vi "Convert Params.vi"(11 "Experiment Parameter Values":T1(array[cluster])) -> (3 "Matlab Param Array":cluster{"Name":string, "Data":variant}[](array[cluster]))   [LabVIEW 2014, in "Matlab API.lvlib"]
uses:
  Matlab API.lvlib
  <vilib>/Utility/error.llb/DialogType.ctl
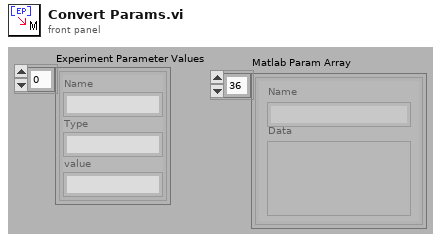
[diagram p1: front panel]
types:
  T1 = cluster{"Name":string, "Type":string, "value":string}[]
  T2 = typedef "DialogType.ctl" = u16
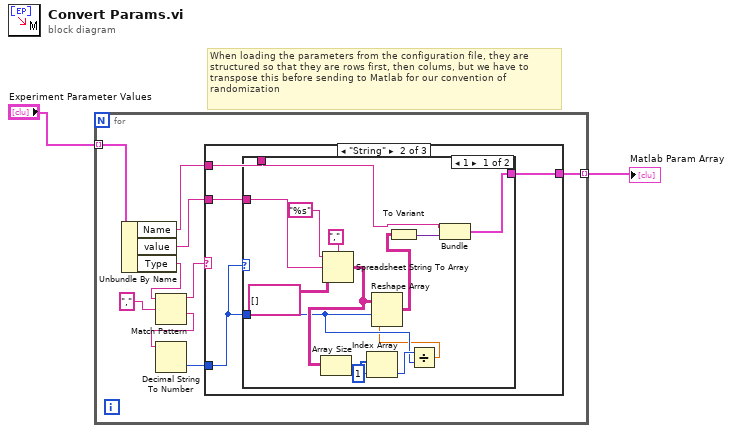
[diagram p0: block diagram]
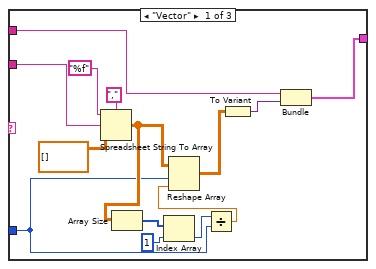
[diagram p2: hidden frame]
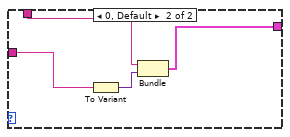
[diagram p3: hidden frame]
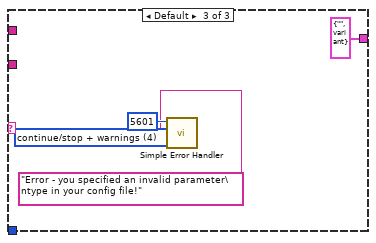
[diagram p4: hidden frame]
diagram:
  # "When loading the parameters from the configuration file, they are \nstructured so that they are rows first, then colums, but we have to \ntranspose this before sending to Matlab for our convention of \nrandomization"
  n1 = for {
    tunnel: "Experiment Parameter Values" -> [w11] mode=indexing
    tunnel: [w8] -> w1 mode=indexing
    n2 = Unbundle By Name(w11) -> ("Name"=w10:string, "value"=w9:string, "Type"=w6:string)
    n3 = Match Pattern(string=w6, regular expression=",") -> (before substring=w5:string, after substring=w4:string)  [unwired: 3 out]
    n4 = Decimal String To Number(string=w4) -> (number=w3:i32)  [unwired: 3 out]
    n5 = case shown="\"String\"" w5 {
      tunnel: w10 -> [w18 w28 _]
      tunnel: w9 -> [w22 w29 _]
      tunnel: [w16 w27 cluster{"Name":string, "Variant":variant} {"Name"="", "Variant"=variant}] -> w8
      tunnel: w3 -> [w12 w26 _]
      frame "Vector" {
        n6 = Spreadsheet String To Array(delimiter (Tab)=",", format string="%f", spreadsheet string=w22, array type (2D Dbl)=dbl[][] []) -> (array=w15:dbl[][])
        n7 = Array Size(array=w15) -> (size(s)=w21:i32[])
        n8 = Index Array(array=w21, index=1) -> (element=w19:i32)
        n9 = Divide(x=w19, y=w12) -> (x/y=w13:dbl)
        n10 = Reshape Array(w15, w12, w13) -> (w14:dbl[][])
        n11 = To Variant(anything=w14) -> (Variant=w17:variant)
        n12 = Bundle("Name"=w18, "Variant"=w17) -> (w16:cluster{"Name":string, "Variant":variant})  [unwired: 1 out]
      }
      frame "String" {
        n13 = case shown="1" w26 {
          tunnel: w29 -> [w40 w47]
          tunnel: w28 -> [w32 w45]
          tunnel: [w31 w44] -> w27
          tunnel: w26 -> [w35 _]
          frame 1 {
            n14 = Spreadsheet String To Array(delimiter (Tab)=",", format string="%s", spreadsheet string=w40, array type (2D Dbl)=string[][] []) -> (array=w39:string[][])
            n15 = Array Size(array=w39) -> (size(s)=w38:i32[])
            n16 = Index Array(array=w38, index=1) -> (element=w36:i32)
            n17 = Divide(x=w36, y=w35) -> (x/y=w34:dbl)
            n18 = Reshape Array(w39, w35, w34) -> (w33:string[][])
            n19 = To Variant(anything=w33) -> (Variant=w30:variant)
            n20 = Bundle("Name"=w32, "Variant"=w30) -> (w31:cluster{"Name":string, "Variant":variant})  [unwired: 1 out]
          }
          frame 0, Default {
            n21 = To Variant(anything=w47) -> (Variant=w46:variant)
            n22 = Bundle("Name"=w45, "Variant"=w46) -> (w44:cluster{"Name":string, "Variant":variant})  [unwired: 1 out]
          }
        }
      }
      frame Default {
        w50 = T2 4 items=["no dialog", "OK message", "continue or stop message", "OK message + warnings", "continue/stop + warnings"] ("type of dialog (OK msg:1)")
        n23 = call <vilib>:"Simple Error Handler.vi"("error code (no error:0)"=5601, "error source (\" \")"="Error - you specified an invalid parameter\ntype in your config file!", "type of dialog (OK msg:1)"=w50) -> ()  [unwired: 1 in, 6 out]
      }
    }
  }
  "Matlab Param Array" <- w1
